vi "Set Up Dialog - Hand Dynamometer.vi"() -> ()   [LabVIEW 2012]
panel:
  in  "GPSN Set Up":bool
  out "Calibration Instructions":string="1. Connect the sensor to your myDAQ as shown in the diagram above.\n\n2. (Optional) Calibrate the Gas Pressure Sensor (GPSN - 100) using the set up instructions below."
  # "iWorx - Hand Dynamometer - Set Up"
  # "Hand Dynamometer"
  # "iWorx"
  # "Sensor"
  # "GPSN - 100"
  # "myDAQ"
  # "Computer"
  # "FT - 220"
  # "Adaptor"
  # "Connection Diagram"
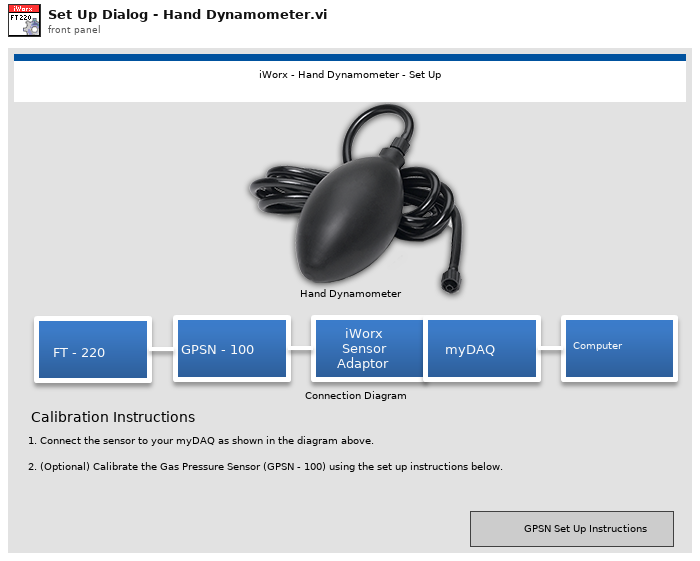
[diagram p1: front panel]
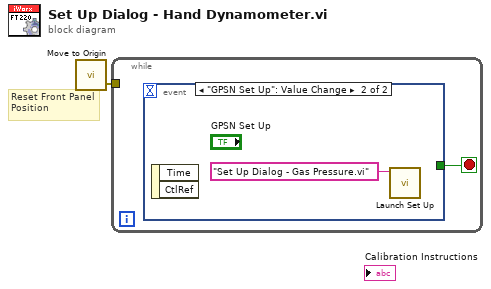
[diagram p0: block diagram]
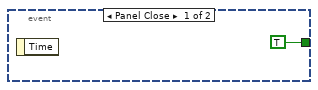
[diagram p2: hidden frame]
diagram:
  # "Reset Front Panel Position"
  n1 = call "Move to Origin.vi"() -> ("Error Out"=w1:errorcluster)  [unwired: 3 in]
  n2 = while {
    tunnel: w1 -> [_]
    stop <- w2 stop-if-true
    n3 = event shown="[1] \"GPSN Set Up\": Value Change" {
      selector: _ -> [_ _]
      dyn-events: _ -> [_ _]
      timeout: _ -> [_ _]
      tunnel: [TRUE _] -> w2
      event Panel Close {
        n4 = event-data() -> ()  [unwired: 1 in, 1 out]
      }
      event "GPSN Set Up": Value Change {
        n5 = event-data() -> ()  [unwired: 1 in, 2 out]
        n6 = call "Launch Set Up.vi"("name or relative path"="Set Up Dialog - Gas Pressure.vi") -> ()  [unwired: 9 in, 2 out]
      }
    }
  }
